vi "parse_string.vi"(8 "bytes per packet":i32, 11 "original content":string) -> (3 "appended array":string[](array[string]))   [LabVIEW 2014]
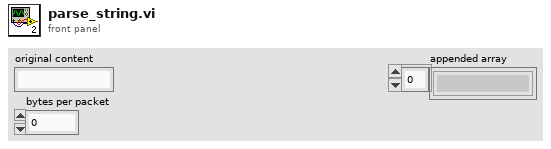
[diagram p1: front panel]
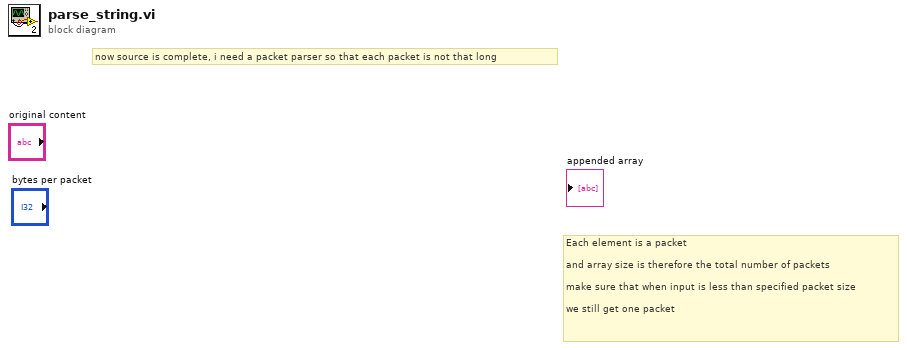
[diagram p0: block diagram]
diagram:
  # "Each element is a packet\n\nand array size is therefore the total number of packets\n\nmake sure that when input is less than specified packet size \n\nwe still get one packet"
  # "now source is complete, i need a packet parser so that each packet is not that long"
